vi "Get_Laser_Cabinet_Status.vi"(8 "error in (no error)":errorcluster, 10 "bytes to read":i32=186, 11 "connection ID":refnum<k5>) -> (0 "error out":errorcluster, 1 "Checksum OK":bool, 2 "output cluster":T1, 3 "connection ID out":refnum<k5>, 4 "Data size":u32)   [LabVIEW 2023]
uses:
  TypeDefs/laser_cabinet_status.ctl
  Globals/Globals.vi
panel:
  out "length 2":i32
  out "Answer":u16
  out "Execution code`":u16
  out "length":i32
  out "data in":string
  out "Data":string
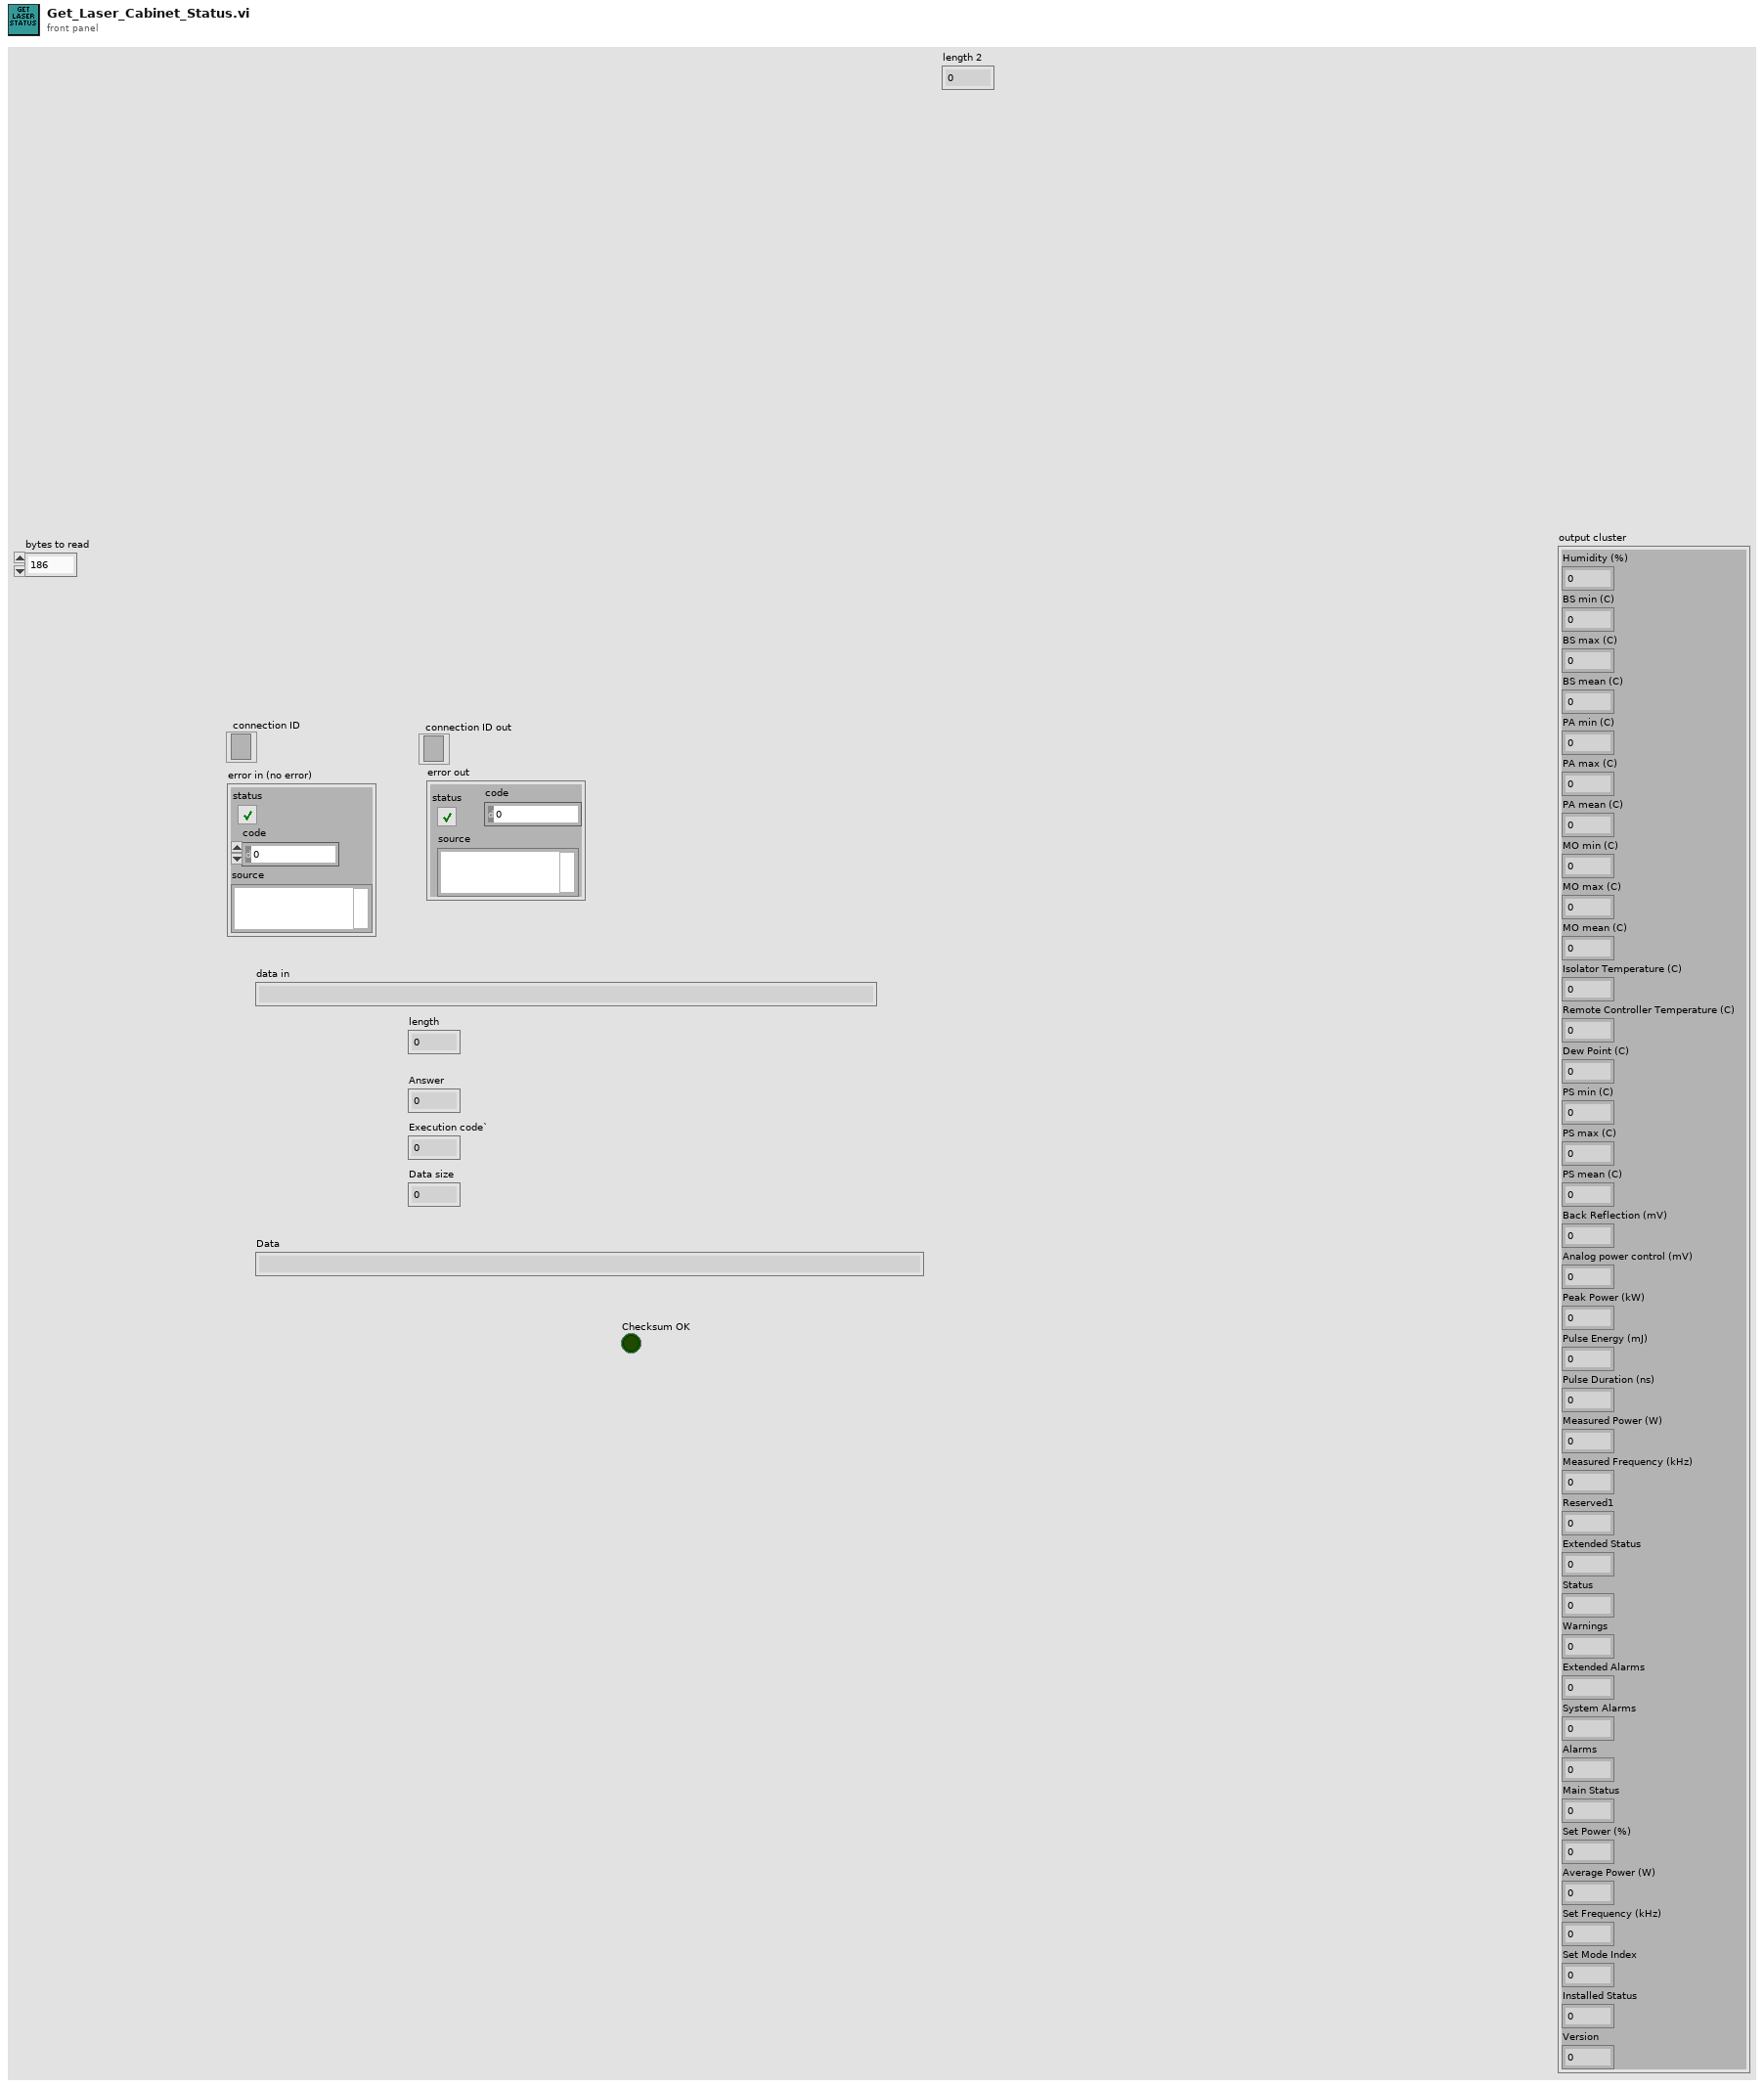
[diagram p1: front panel]
types:
  T1 = typedef "laser_cabinet_status.ctl" = cluster{"Version":u16, "Installed Status":u32, "Set Mode Index":u16, "Set Frequency (kHz)":sgl, "Average Power (W)":sgl, "Set Power (%)":sgl, "Main Status":u32, "Alarms":u32, "System Alarms":u32, "Extended Alarms":u32, "Warnings":u32, "Status":u32, "Extended Status":u32, "Reserved1":u16, "Measured Frequency (kHz)":sgl, "Pulse Duration (ns)":u32, "Measured Power (W)":sgl, "Pulse Energy (mJ)":sgl, "Peak Power (kW)":sgl, "Analog power control (mV)":sgl, "Back Reflection (mV)":sgl, "PS mean (C)":sgl, "PS max (C)":sgl, "PS min (C)":sgl, "Dew Point (C)":sgl, "Remote Controller Temperature (C)":sgl, "Isolator Temperature (C)":sgl, "MO mean (C)":sgl, "MO max (C)":sgl, "MO min (C)":sgl, "PA mean (C)":sgl, "PA max (C)":sgl, "PA min (C)":sgl, "BS mean (C)":sgl, "BS max (C)":sgl, "BS min (C)":sgl, "Humidity (%)":sgl}
  T2 = enum16{"big-endian, network order", "native, host order", "little-endian"}
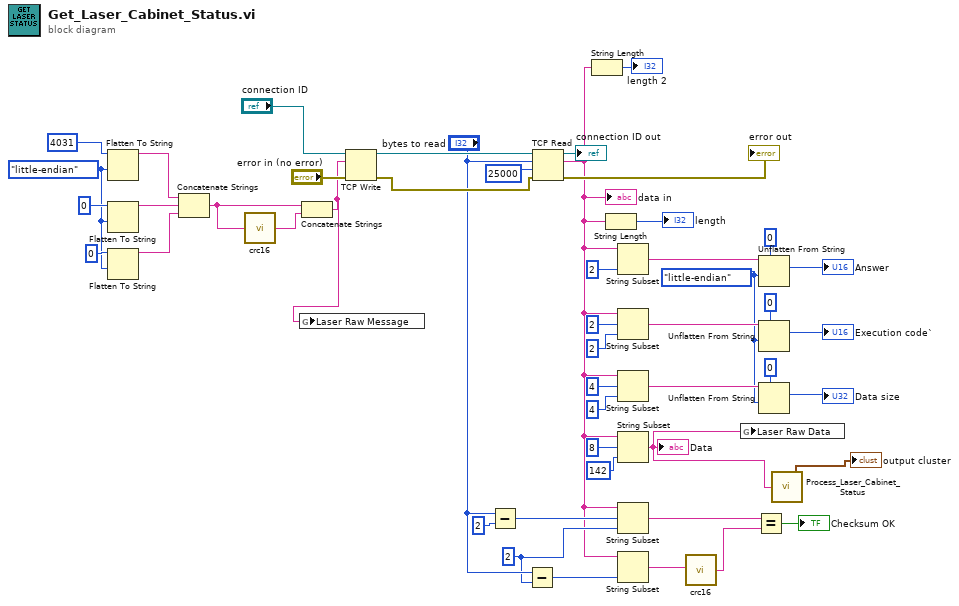
[diagram p0: block diagram]
diagram:
  w16 = T2."little-endian" ("byte order (0:big-endian, network order)")
  w24 = T2."little-endian" ("byte order (0:big-endian, network order)")
  w35 = 2 ("length (rest)")
  n1 = Flatten To String(anything=u16 4031 ("Command"), byte order (0:big-endian, network order)=w24) -> (data string=w30:string)  [unwired: 2 in, 2 out]
  n2 = Flatten To String(anything=u16 0, byte order (0:big-endian, network order)=w24) -> (data string=w29:string)  [unwired: 2 in, 2 out]
  n3 = Flatten To String(anything=u32 0 ("Datasize"), byte order (0:big-endian, network order)=w24) -> (data string=w28:string)  [unwired: 2 in, 2 out]
  n4 = Concatenate Strings(w30, w29, w28) -> (w12:string)
  n5 = call "crc16.vi"("string"=w12) -> ("string 2"=w13:string)
  n6 = Concatenate Strings(w12, w13) -> (w1:string)
  n7 = global write "Globals.vi" "Laser Raw Message"(w1) -> ()
  n8 = TCP Write(connection ID="connection ID", data in=w1, error in (no error)="error in (no error)") -> (connection ID out=w48:refnum<k5>, error out=w46:errorcluster)  [unwired: 1 in, 1 out]
  n9 = Subtract(x="bytes to read", y=2 ("offset (0)")) -> (x-y=w38:i32)
  n10 = Subtract(x="bytes to read", y=w35) -> (x-y=w34:i32)
  n11 = TCP Read(connection ID=w48, bytes to read="bytes to read", error in (no error)=w46, 9:25000 ("timeout ms (25000)")) -> (connection ID out=→"connection ID out":refnum<k5>, data out=w4:string, error out=→"error out":errorcluster)  [unwired: 1 in]
  "data in" <- w4
  n12 = String Length(string=w4) -> (length=→"length 2":i32)
  n13 = String Length(string=w4) -> (length=→"length":i32)
  n14 = String Subset(string=w4, length (rest)=2 ("length (rest)")) -> (substring=w22:string)  [unwired: 1 in]
  n15 = String Subset(string=w4, offset (0)=2, length (rest)=2 ("length (rest)")) -> (substring=w20:string)
  n16 = String Subset(string=w4, offset (0)=4, length (rest)=4 ("length (rest)")) -> (substring=w17:string)
  n17 = String Subset(string=w4, offset (0)=8, length (rest)=142 ("length (rest)")) -> (substring=w2:string)
  "Data" <- w2
  n18 = String Subset(string=w4, offset (0)=w38, length (rest)=w35) -> (substring=w37:string)
  n19 = String Subset(string=w4, length (rest)=w34) -> (substring=w11:string)  [unwired: 1 in]
  n20 = call "crc16.vi"("string"=w11) -> ("string 2"=w10:string)
  n21 = global write "Globals.vi" "Laser Raw Data"(w2) -> ()
  n22 = Equal?(x=w37, y=w10) -> (x = y?=→"Checksum OK":bool)
  n23 = Unflatten From String(type=u16 0, binary string=w22, byte order (0:big-endian, network order)=w16) -> (value=→"Answer":u16)  [unwired: 2 in, 2 out]
  n24 = Unflatten From String(type=u16 0, binary string=w20, byte order (0:big-endian, network order)=w16) -> (value=→"Execution code`":u16)  [unwired: 2 in, 2 out]
  n25 = Unflatten From String(type=u32 0, binary string=w17, byte order (0:big-endian, network order)=w16) -> (value=→"Data size":u32)  [unwired: 2 in, 2 out]
  n26 = call "Process_Laser_Cabinet_Status.vi"("Data"=w2) -> ("output cluster 2"=→"output cluster":T1)
